vi "(SubVI) Fitting Sine Wave_YCC.vi"(6 "Start Position (um)":dbl, 8 "f_drive (Hz)":dbl, 9 "Amplitude, A (nm)":dbl, 10 "Position array (um)":dbl[](array[numeric]), 11 "Time array (s)":dbl[](array[numeric])) -> (0 "True Amplitude, A (nm)":dbl, 1 "best nonlinear fit for cut position":dbl[](array[numeric]), 2 "Cut-Position Array (um)":dbl[](array[numeric]), 3 "Cut-Time Array (s)":dbl[](array[numeric]), 4 "True f_drive (Hz)":dbl, 5 "best fit parameters":dbl[](array[numeric]))   [LabVIEW 2014]
uses:
  <vilib>/gmath/NumericalOptimization/Nonlinear Curve Fit LM formula string.vi
  <vilib>/gmath/NI_Gmath.lvlib
panel:
  out "Initial guess":dbl[](array[numeric])
  out "A scaling":dbl
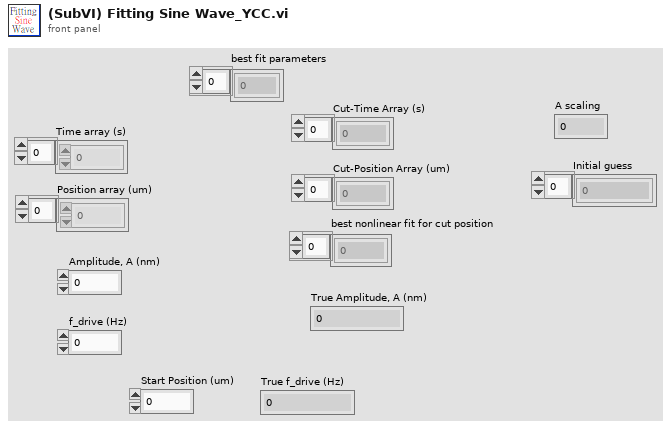
[diagram p1: front panel]
types:
  T1 = cluster{"model":string, "Parameters":string[], "x":string}
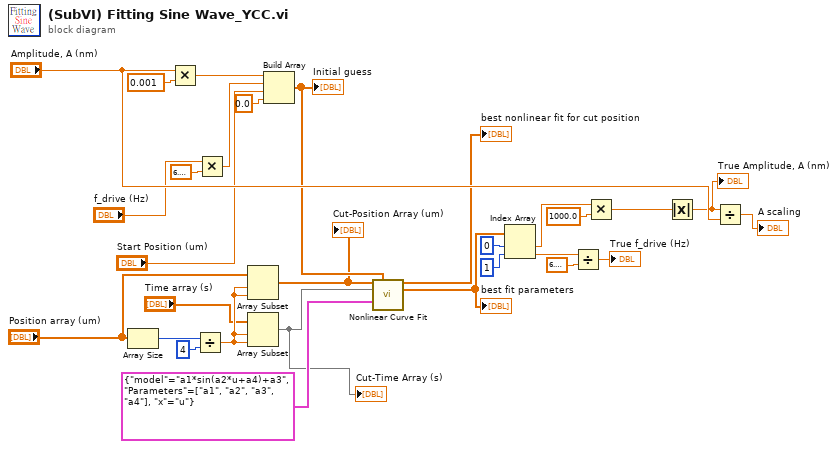
[diagram p0: block diagram]
diagram:
  n1 = Array Size(array="Position array (um)") -> (size(s)=w7:i32)
  n2 = Multiply(x="Amplitude, A (nm)", y=0.001) -> (x*y=w23:dbl)
  n3 = Divide(x=w7, y=4) -> (x/y=w5:dbl)
  n4 = Multiply(x="f_drive (Hz)", y=6.283185307179586) -> (x*y=w27:dbl)
  n5 = Array Subset(array="Position array (um)", index=w5, length=w5) -> (w2:dbl[])
  "Cut-Position Array (um)" <- w2
  n6 = Array Subset(array="Time array (s)", index=w5, length=w5) -> (w1:dbl[])
  "Cut-Time Array (s)" <- w1
  n7 = Build Array(w23, w27, "Start Position (um)", 0.0 ("element")) -> (w21:dbl[])
  "Initial guess" <- w21
  n8 = call-poly <vilib>:"Nonlinear Curve Fit.vi"("Y"=w2, "initial parameters"=w21, "X"=w1, "model description"=T1 {"model"="a1*sin(a2*u+a4)+a3", "Parameters"=["a1", "a2", "a3", "a4"], "x"="u"}) -> ("best nonlinear fit"=→"best nonlinear fit for cut position":dbl[], "best fit parameters"=w8:dbl[])  [unwired: 7 in, 3 out]
  "best fit parameters" <- w8
  n9 = Index Array(array=w8, index #1=0 ("index"), index #2=1 ("index")) -> (element #1=w14:dbl, element #2=w15:dbl)
  n10 = Divide(x=w15, y=6.283185307179586) -> (x/y=→"True f_drive (Hz)":dbl)
  n11 = Multiply(x=w14, y=1000.0) -> (x*y=w17:dbl)
  n12 = Absolute Value(x=w17) -> (abs(x)=w18:dbl)
  "True Amplitude, A (nm)" <- w18
  n13 = Divide(x=w18, y="Amplitude, A (nm)") -> (x/y=→"A scaling":dbl)
